vi "Board_Type_Strings.vi"(0 "Board type":T1) -> (1 "Board String":string, 2 "Acquisition VI Name":string)   [LabVIEW 2011]
uses:
  Board_Types.ctl
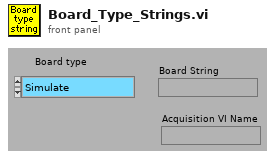
[diagram p1: front panel]
types:
  T1 = typedef "Board_Types.ctl" = enum16{"Simulate", "Local ADAM", "Server ADAM", "NI-DAQmx", "NI-DAQmxBase", "ADC488", "DT LV-link"}
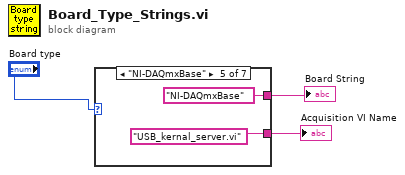
[diagram p0: block diagram]
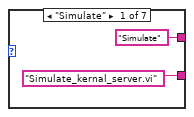
[diagram p2: hidden frame]
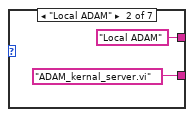
[diagram p3: hidden frame]
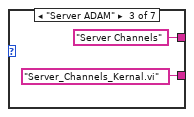
[diagram p4: hidden frame]
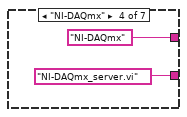
[diagram p5: hidden frame]
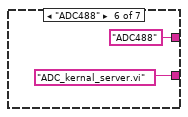
[diagram p6: hidden frame]
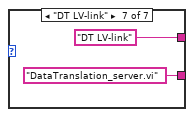
[diagram p7: hidden frame]
diagram:
  n1 = case shown="\"NI-DAQmxBase\"" "Board type" {
    tunnel: ["Simulate" "Local ADAM" "Server Channels" "NI-DAQmx" "NI-DAQmxBase" "ADC488" "DT LV-link"] -> w2
    tunnel: ["Simulate_kernal_server.vi" "ADAM_kernal_server.vi" "Server_Channels_Kernal.vi" "NI-DAQmx_server.vi" "USB_kernal_server.vi" "ADC_kernal_server.vi" "DataTranslation_server.vi"] -> w1
    frame "Simulate" {
    }
    frame "Local ADAM" {
    }
    frame "Server ADAM" {
    }
    frame "NI-DAQmx" {
    }
    frame "NI-DAQmxBase" {
    }
    frame "ADC488" {
    }
    frame "DT LV-link" {
    }
  }
  "Board String" <- w2
  "Acquisition VI Name" <- w1
